vi "Global Load.vi"(8 "error in (no error)":errorcluster, 10 "Startup.ini":path, 11 "Global in":refnum<k1>) -> (0 "error out":errorcluster, 1 "Apps":cluster{"Instances":T1[]}[](array[cluster]), 2 "App Names":string[](array[string]), 3 "Global out":refnum<k1>)   [LabVIEW 2018, in "Shared.lvlib"]
uses:
  Shared.lvlib
  Controls/Global.ctl
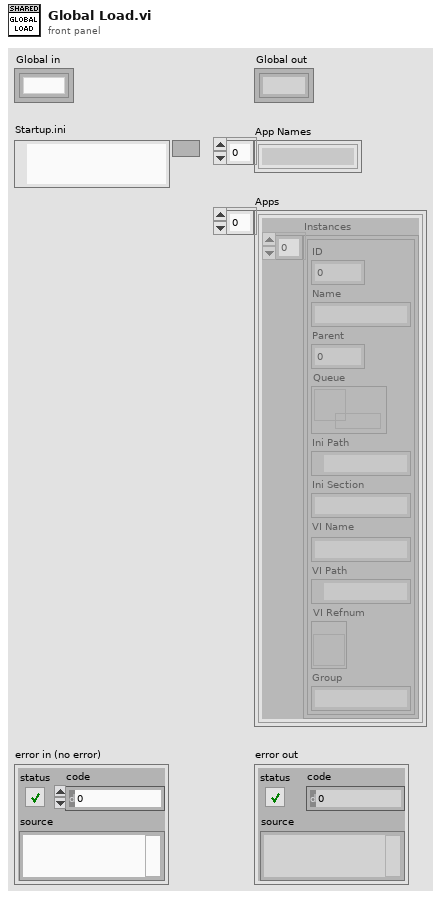
[diagram p1: front panel]
types:
  T1 = typedef "Shared.lvlib/Global.ctl" = cluster{"ID":i32, "Name":string, "Parent":i32, "Queue":refnum<queue>, "Ini Path":path, "Ini Section":string, "VI Name":string, "VI Path":path, "VI Refnum":refnum<vi>, "Group":string}
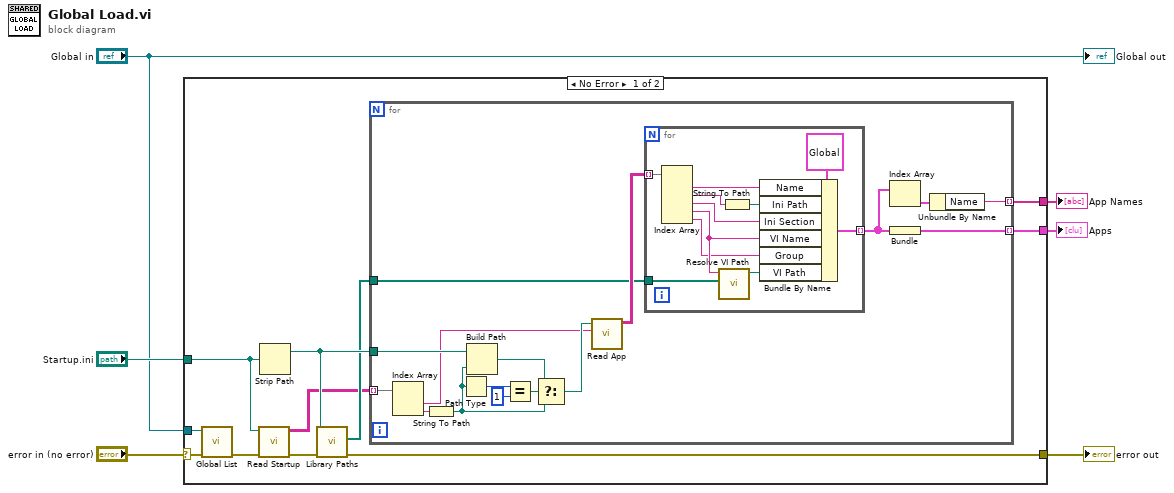
[diagram p0: block diagram]
diagram:
  n1 = case shown="No Error" "error in (no error)" {
    selector: "error in (no error)" -> [w17 w45]
    tunnel: [w15 w45] -> w6
    tunnel: "Startup.ini" -> [w10 _]
    tunnel: "Global in" -> [w16 _]
    tunnel: [w8 _] -> w2
    tunnel: [w7 _] -> w1
    frame No Error {
      n2 = call "Global List.vi"("error in (no error)"=w17, "Global in"=w16) -> ("error out"=w12:errorcluster)  [unwired: 7 in, 2 out]
      n3 = call "Read Startup.vi"("error in (no error)"=w12, "Path (*.ini)"=w10) -> ("error out"=w11:errorcluster, "Name,Path"=w9:string[][])  [unwired: 8 in]
      n4 = Strip Path(path=w10) -> (stripped path=w14:path)  [unwired: 1 out]
      n5 = call "Library Paths.vi"("error in (no error)"=w11, "Base Dir in"=w14) -> ("error out"=w15:errorcluster, "Packed Libraries (.lvlibp)"=w13:path[])  [unwired: 6 in, 2 out]
      n6 = for {
        tunnel: w14 -> [w28]
        tunnel: w13 -> [w22]
        tunnel: w9 -> [w26] mode=indexing
        tunnel: [w21] -> w8 mode=indexing
        tunnel: [w18] -> w7 mode=indexing
        n7 = Index Array(array=w26) -> (element #1=w25:string, element #2=w24:string)  [unwired: 2 in]
        n8 = String To Path(string=w24) -> (path=w30:path)
        n9 = Path Type(1:w30) -> (0:w33:i16)
        n10 = Build Path(base path=w28, name or relative path=w30) -> (appended path=w31:path)
        n11 = Equal?(x=w33, y=i16 1) -> (x = y?=w32:bool)
        n12 = Select(t=w31, s=w32, f=w30) -> (s? t:f=w27:path)
        n13 = call "Read App.vi"("App Name"=w25, "Path (*.ini)"=w27) -> ("Name,Path,Section,VI,Group"=w23:string[][])  [unwired: 8 in, 1 out]
        n14 = for {
          tunnel: w23 -> [w44] mode=indexing
          tunnel: w22 -> [w36]
          tunnel: [w34] -> w20 mode=indexing
          n15 = Index Array(array=w44) -> (element #1=w42:string, element #2=w41:string, element #3=w39:string, element #4=w38:string, element #5=w35:string)  [unwired: 5 in]
          n16 = call "Resolve VI Path.vi"("Library Paths (.lvlibp, .lvlib)"=w36, "Qualified Name (lvlibp|lvlib[:vi])"=w38) -> ("VI Path"=w37:path)  [unwired: 7 in, 2 out]
          n17 = String To Path(string=w41) -> (path=w40:path)
          n18 = Bundle By Name(cluster=T1 {"ID"=0, "Name"="", "Parent"=0, "Queue"=refnum, "Ini Path"=path "", "Ini Section"="", "VI Name"="", "VI Path"=path "", "VI Refnum"=refnum, "Group"=""} ("Global"), "Name"=w42, "Ini Path"=w40, "Ini Section"=w39, "VI Name"=w38, "Group"=w35, "VI Path"=w37) -> (w34:T1)
        }
        n19 = Index Array(array=w20) -> (element=w19:T1)  [unwired: 1 in]
        n20 = Bundle(w20) -> (w21:cluster{T1[]})  [unwired: 1 in]
        n21 = Unbundle By Name(w19) -> ("Name"=w18:string)
      }
    }
    frame Error {
    }
  }
  "error out" <- w6
  "Apps" <- w2
  "App Names" <- w1
  "Global out" <- "Global in"
